vi "ApproveYCoord (SubVI).vi"(8 "Yhigh":dbl, 9 "Ylow":dbl, 11 "Go to Y":dbl) -> (3 "Pass Y?":bool)   [LabVIEW 2016]
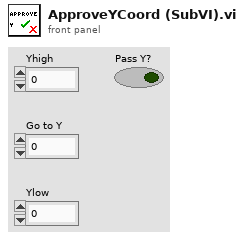
[diagram p1: front panel]
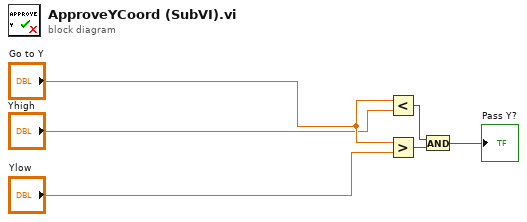
[diagram p0: block diagram]
diagram:
  n1 = Less?(x="Go to Y", y="Yhigh") -> (x < y?=w4:bool)
  n2 = Greater?(x="Go to Y", y="Ylow") -> (0:w5:bool)
  n3 = And(x=w4, y=w5) -> (x .and. y?=→"Pass Y?":bool)
